vi "GUI.vi"() -> ()   [LabVIEW 2019]
panel:
  in  "Expiration Pause\nDuration":dbl(slide)=1.0204081632653061 scale=0.0..5.0
  in  "Expiration Pause\nTarget Pressure":dbl(slide)=5.1020408163265305 scale=0.0..50.0
  in  "Expiration Flow \nDuration":dbl(slide)=1.0204081632653061 scale=0.0..5.0
  in  "Expiration Flow \nTarget Pressure":dbl(slide)=5.1020408163265305 scale=0.0..50.0
  in  "Inspiration Pause\nDuration":dbl(slide)=0.9693877551020409 scale=0.0..5.0
  in  "Inspiration Pause\nTarget Pressure":dbl(slide)=15.816326530612246 scale=0.0..50.0
  in  "Inspriation Flow \nDuration":dbl(slide)=1.4285714285714286 scale=0.0..5.0
  in  "Inspiration Flow \nTarget Pressure":dbl(slide)=20.918367346938776 scale=0.0..50.0
  out "Pressure":dynamicdata(graph)
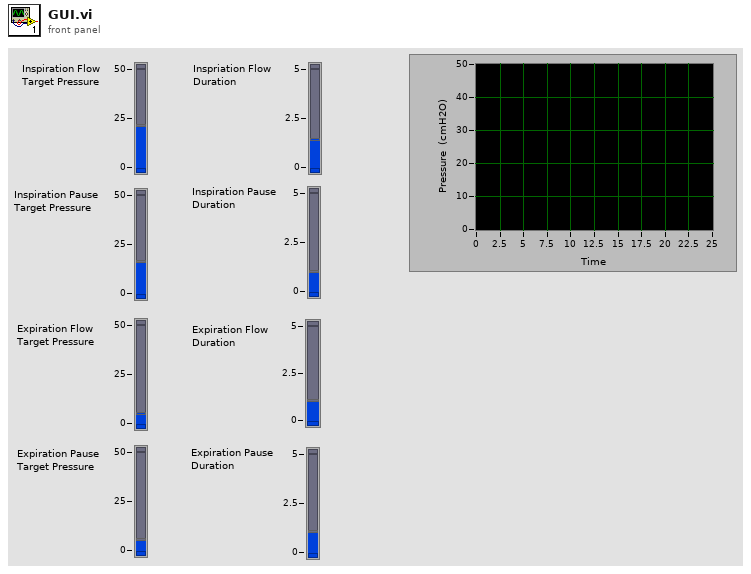
[diagram p1: front panel]
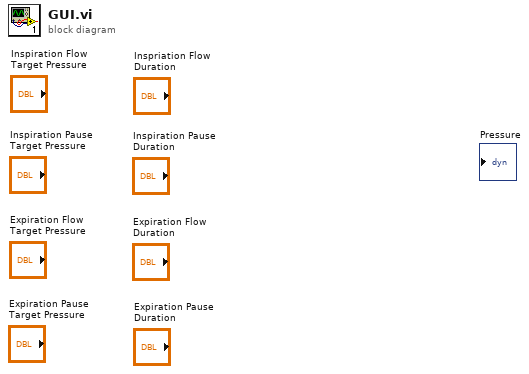
[diagram p0: block diagram]
diagram:
